vi "TagCheck.vi"(10 "Tags":string[](array[string]), 11 "?":cluster{"Folder Path":path, string[]}) -> (2 "Good?":bool, 3 "Path out":path)   [LabVIEW 2022 SP3]
panel:
  out "Array":bool[][](array[boolean])
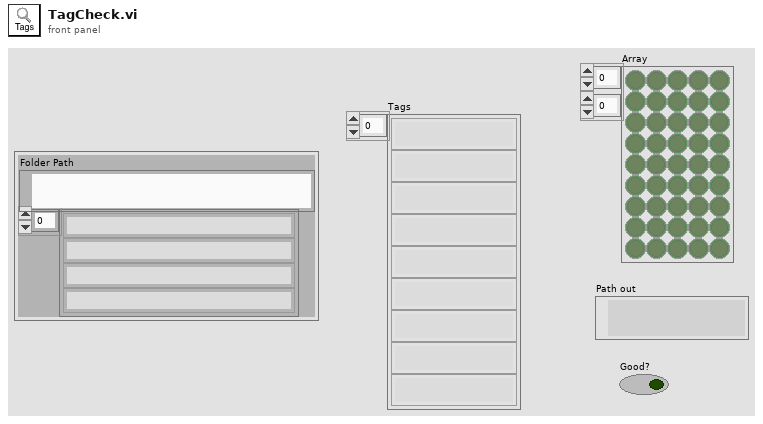
[diagram p1: front panel]
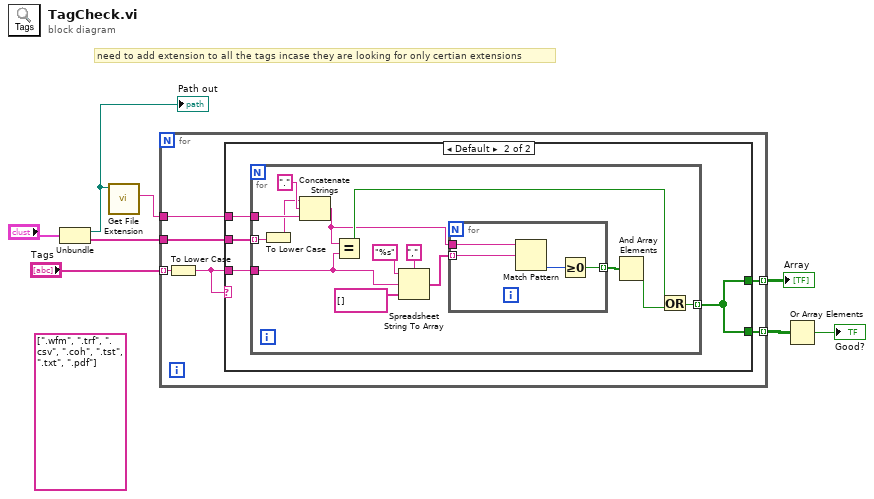
[diagram p0: block diagram]
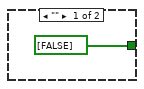
[diagram p2: hidden frame]
diagram:
  (unwired) string[] [".wfm", ".trf", ".csv", ".coh", ".tst", ".txt", ".pdf"] ("array type (2D Dbl)")
  # "need to add extension to all the tags incase they are looking for only certian extensions"
  n1 = Unbundle("?") -> ("Folder Path"=w3:path, w4:string[])
  "Path out" <- w3
  n2 = call <vilib>:"Get File Extension.vi"("file"=w3) -> ("lowercase file extension"=w2:string)  [unwired: 6 in, 4 out]
  n3 = for {
    tunnel: "Tags" -> [w10] mode=indexing
    tunnel: [w14] -> w7 mode=indexing
    tunnel: w4 -> [w13]
    tunnel: w2 -> [w12]
    tunnel: [w11] -> w1 mode=indexing
    n4 = To Lower Case(string=w10) -> (all lower case string=w9:string)
    n5 = case shown="Default" w9 {
      tunnel: w9 -> [_ w19]
      tunnel: [bool[] [FALSE] w16] -> w14
      tunnel: w13 -> [_ w18]
      tunnel: w12 -> [_ w17]
      tunnel: [_ w16] -> w11
      frame "" {
      }
      frame Default {
        n6 = for {
          tunnel: w19 -> [w28]
          tunnel: [w26] -> w16 mode=indexing
          tunnel: w18 -> [w21] mode=indexing
          tunnel: w17 -> [w23]
          n7 = To Lower Case(string=w21) -> (all lower case string=w20:string)
          n8 = Concatenate Strings(w20, "." ("string"), w23) -> (w22:string)
          n9 = Equal?(x=w22, y=w28) -> (x = y?=w27:bool)
          n10 = Spreadsheet String To Array(delimiter (Tab)=",", format string="%s", spreadsheet string=w28, array type (2D Dbl)=string[] []) -> (array=w31:string[])
          n11 = for {
            tunnel: w31 -> [w34] mode=indexing
            tunnel: w22 -> [w36]
            tunnel: [w35] -> w33 mode=indexing
            n12 = Match Pattern(string=w36, regular expression=w34) -> (offset past match=w37:i32)  [unwired: 1 in, 3 out]
            n13 = Greater Or Equal To 0?(x=w37) -> (x >= 0?=w35:bool)
          }
          n14 = And Array Elements ("And Array")(Boolean array=w33) -> (logical AND=w25:bool)
          n15 = Or(x=w27, y=w25) -> (x .or. y?=w26:bool)
        }
      }
    }
  }
  "Array" <- w1
  n16 = Or Array Elements(Boolean array=w7) -> (logical OR=→"Good?":bool)
